vi "Loop_HW.vi"   [LabVIEW 2017, in "Gear.lvlib"]
uses:
  Gear.lvlib
  <vilib>/Rock Robotics/WPI/Solenoid/WPI_SolenoidChannel.ctl
  <vilib>/Rock Robotics/WPI/Solenoid/WPI_SolenoidOpenDouble.vi
  Globals/Global_STOP.vi
  Global_GearPistonsCTRL.vi
  <vilib>/Rock Robotics/WPI/Solenoid/WPI_SolenoidSetEnum.vi
types:
  T1 = typedef "WPI_SolenoidChannel.ctl" = enum8{"Solenoid 0", "Solenoid 1", "Solenoid 2", "Solenoid 3", "Solenoid 4", "Solenoid 5", "Solenoid 6", "Solenoid 7", "Invalid"}
  T2 = typedef "WPI_SolenoidDevRef.ctl" = cluster{"DevStatus":errorcluster, "Pneumatics Control Module":u8, "Forward Solenoid Channel":T1, "Reverse Solenoid Channel":T1}
  T3 = typedef "WPI_CompressorDevRef.ctl" = cluster{"DevStatus":errorcluster, "Pneumatics Control Module":u8}
  T4 = typedef "WPI_SolenoidValue.ctl" = enum16{"Off", "On", "Forward", "Reverse"}
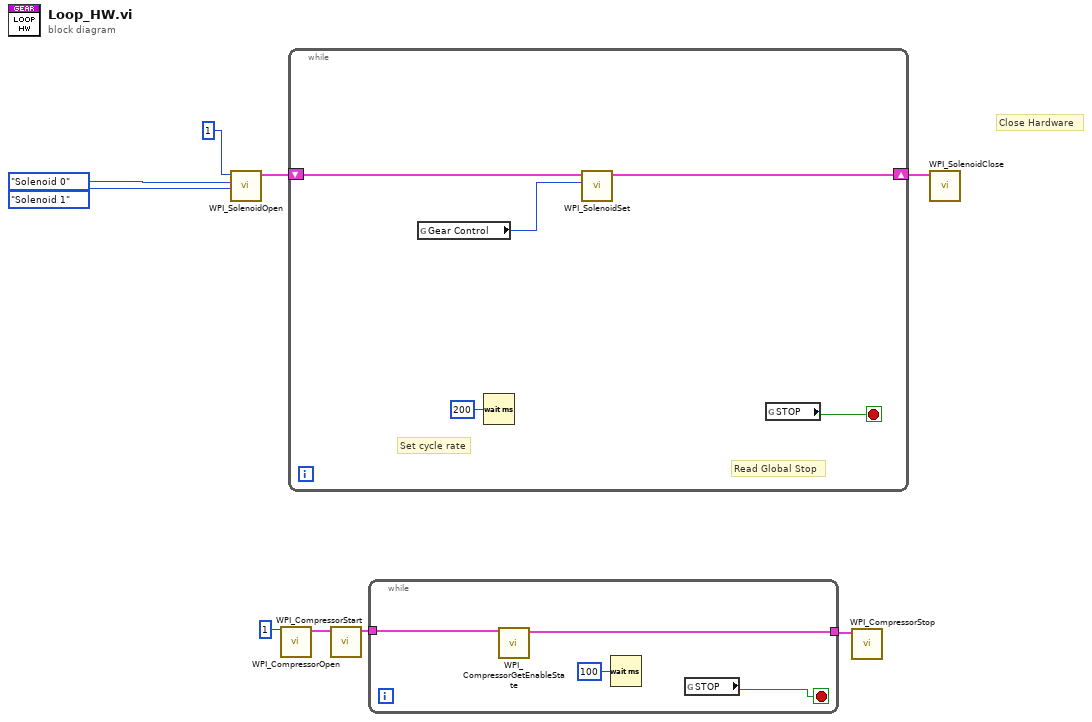
[diagram p0: block diagram]
diagram:
  # "Close Hardware"
  n1 = call-poly <vilib>:"WPI_SolenoidOpen.vi"("Reverse Solenoid Channel"=WPI_SolenoidChannel."Solenoid 1", "Forward Solenoid Channel"=WPI_SolenoidChannel."Solenoid 0", "Pneumatics Control Module (0)"=u8 1) -> ("SolenoidDevRef"=w9:T2)  [unwired: 7 in, 1 out]
  n2 = call <vilib>:"WPI_CompressorOpen.vi"("Pneumatics Control Module (0)"=u8 1) -> ("CompressorDevRef"=w4:T3)  [unwired: 13 in, 1 out]
  n3 = while {
    shift-right: [w11] -> w7
    shift-left: w9 -> [w12]
    stop <- w13 stop-if-true
    # "Read Global Stop"
    # "Set cycle rate"
    n4 = global read "Global_GearPistonsCTRL.vi" "Gear Control"() -> (w10:T4)
    n5 = Wait (ms)(milliseconds to wait=u32 200) -> ()  [unwired: 1 out]
    n6 = call-poly <vilib>:"WPI_SolenoidSet.vi"("Value"=w10, "SolenoidDevRef"=w12) -> ("SolenoidDevRef"=w11:T2)  [unwired: 8 in, 1 out]
    n7 = global read "Global_Stop.vi" "STOP"() -> (w13:bool)
  }
  n8 = call <vilib>:"WPI_CompressorStart.vi"("CompressorDevRef"=w4) -> ("CompressorDevRef"=w3:T3)  [unwired: 1 in, 9 out]
  n9 = while {
    tunnel: w3 -> [w18]
    tunnel: [w17] -> w1
    stop <- w15 stop-if-true
    n10 = call <vilib>:"WPI_CompressorGetEnableState.vi"("CompressorDevRef"=w18) -> ("CompressorDevRef"=w17:T3)  [unwired: 1 in, 9 out]
    n11 = Wait (ms)(milliseconds to wait=u32 100) -> ()  [unwired: 1 out]
    n12 = global read "Global_STOP.vi" "STOP"() -> (w15:bool)
  }
  n13 = call <vilib>:"WPI_CompressorStop.vi"("CompressorDevRef"=w1) -> ()  [unwired: 1 in, 10 out]
  n14 = call <vilib>:"WPI_SolenoidClose.vi"("SolenoidDevRef"=w7) -> ()  [unwired: 10 in, 1 out]
